vi "Handle Command.vi"(8 "error in (no error)":errorcluster, 9 "Data":variant, 10 "Command":string, 11 "Example Instrument in":refnum<class "Instrument.Element2.lvclass">) -> (0 "error out":errorcluster, 1 "Processed Data":variant, 2 "Command":string, 3 "Example Instrument out":refnum<class "Instrument.Element2.lvclass">)   [LabVIEW 2019, in "Instrument.Element2.lvclass"]
uses:
  Instrument.Element2.lvclass
  537bce52-1556-4e80-bd1c-c7a4a9f398bb.vi
  29a2691b-054e-4a4e-beb1-253e02bda3af.vi
  59852270-7c69-4675-bfeb-e3c756fddd99.vi
  537bce52-1556-4e80-bd1c-c7a4a9f398bb.vi/cb4d4a81-1a0b-4a34-ba5f-4adbbd4c364d.vi
  537bce52-1556-4e80-bd1c-c7a4a9f398bb.vi/c7ebcf92-25f2-4bb9-8687-30e4771393b5.vi
  29a2691b-054e-4a4e-beb1-253e02bda3af.vi/ce10c08f-31f2-4d71-8816-27111e331727.vi
  29a2691b-054e-4a4e-beb1-253e02bda3af.vi/b0a342ce-c0c6-4751-9e7d-832a740cbd2c.vi
  59852270-7c69-4675-bfeb-e3c756fddd99.vi/d4115e51-0f20-4ace-a191-9b88fbaefa4e.vi
  59852270-7c69-4675-bfeb-e3c756fddd99.vi/2ebf8451-a15d-4a57-978f-c6fd804eee3c.vi
  <vilib>/Utility/Data Type/Get Type Information.vi
  <vilib>/JDP Science/JSONtext/JSON text to Variant.vi
  <vilib>/JDP Science/JSONtext/LVClass Serializer/JSONtext LVClass Serializer.lvclass
  <userlib>/LevyLab/Instrument Framework/Instrument Types/VSource/Instrument.VSource.lvclass
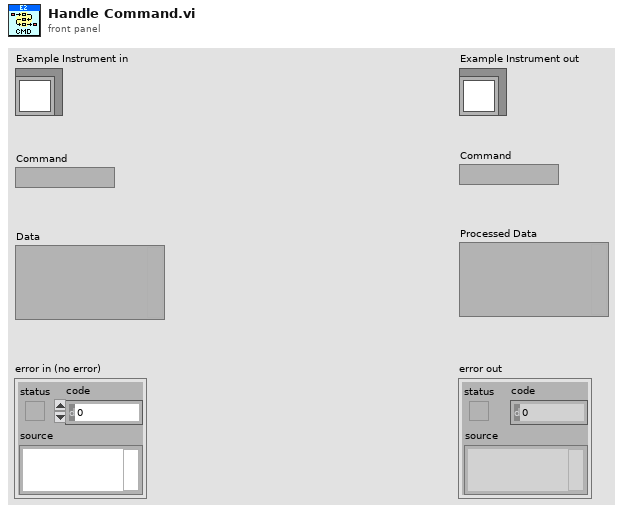
[diagram p1: front panel]
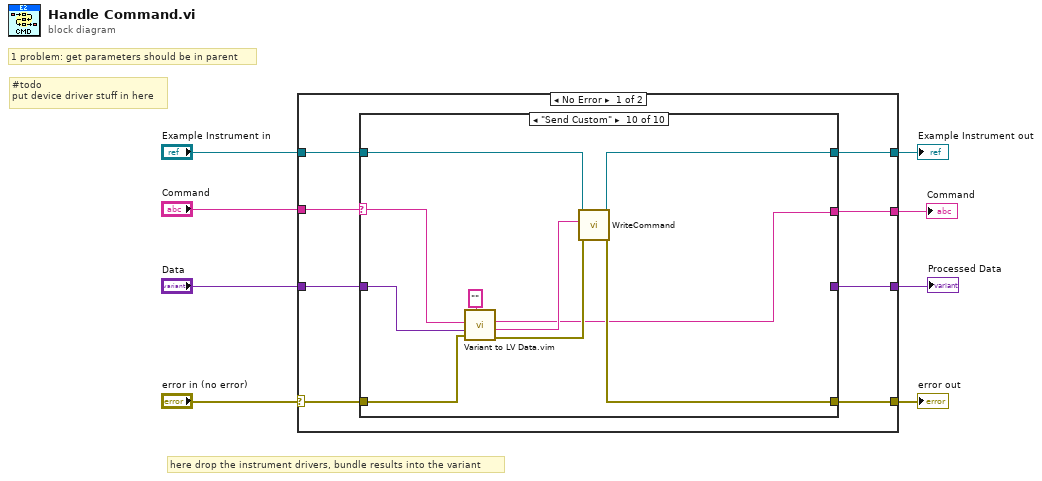
[diagram p0: block diagram]
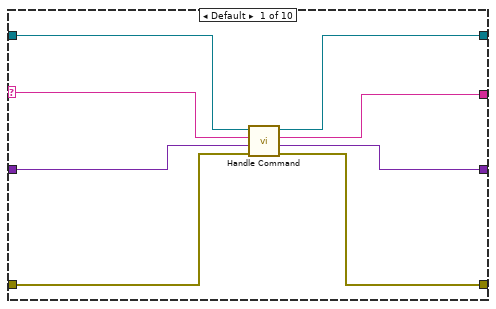
[diagram p2: hidden frame]
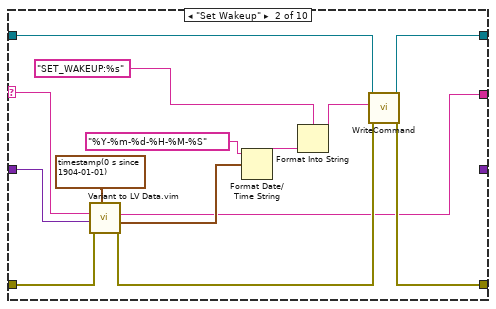
[diagram p3: hidden frame]
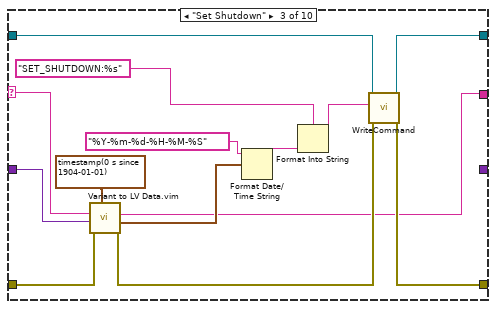
[diagram p4: hidden frame]
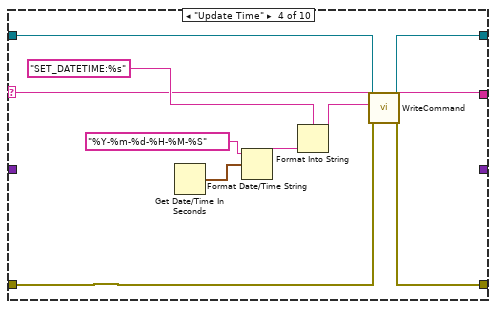
[diagram p5: hidden frame]
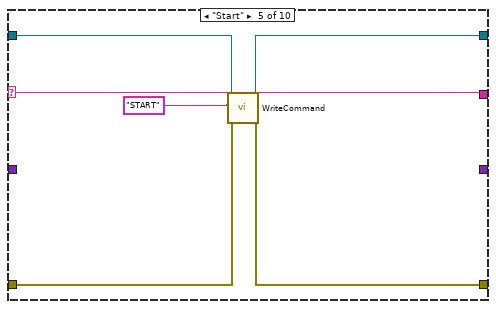
[diagram p6: hidden frame]
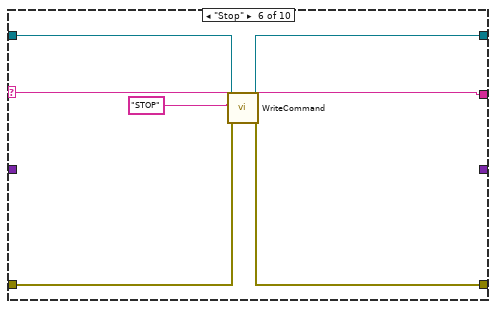
[diagram p7: hidden frame]
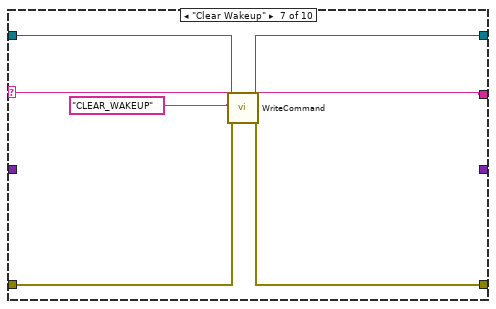
[diagram p8: hidden frame]
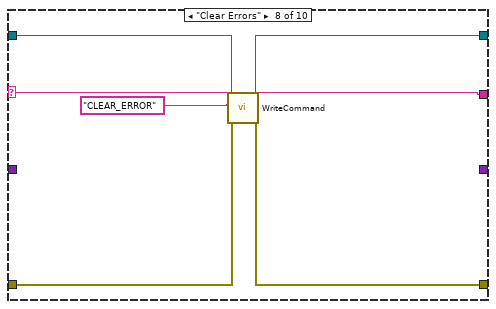
[diagram p9: hidden frame]
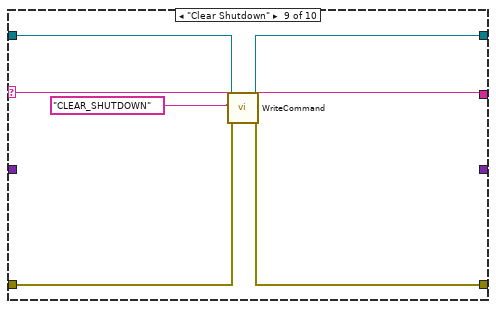
[diagram p10: hidden frame]
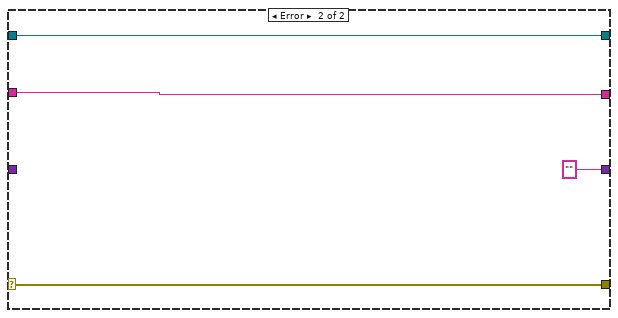
[diagram p11: hidden frame]
diagram:
  # "here drop the instrument drivers, bundle results into the variant"
  # "1 problem: get parameters should be in parent"
  # "#todo\nput device driver stuff in here"
  n1 = case shown="No Error" "error in (no error)" {
    selector: "error in (no error)" -> [w12 w106]
    tunnel: [w10 w106] -> w6
    tunnel: [w14 w105] -> w5
    tunnel: "Example Instrument in" -> [w15 w105]
    tunnel: "Command" -> [w16 w103]
    tunnel: [w13 "" ("String")] -> w3
    tunnel: "Data" -> [w11 _]
    tunnel: [w9 w103] -> w1
    frame No Error {
      n2 = case shown="\"Send Custom\"" w16 {
        selector: w16 -> [w24 w29 w43 w53 w63 w69 w75 w81 w87 w98]
        tunnel: w15 -> [w21 w38 w52 w62 w68 w74 w80 w86 w92 w102]
        tunnel: [w18 w37 w51 w61 w67 w73 w79 w85 w91 w101] -> w14
        tunnel: [w20 _ _ _ _ _ _ _ _ _] -> w13
        tunnel: w12 -> [w22 w28 w42 w55 w65 w71 w77 w83 w89 w97]
        tunnel: w11 -> [w23 w32 w46 _ _ _ _ _ _ w99]
        tunnel: [w19 w26 w40 w56 w66 w72 w78 w84 w90 w100] -> w10
        tunnel: [w17 w25 w39 w53 w63 w69 w75 w81 w87 w93] -> w9
        frame Default {
          n3 = call-parent "Handle Command.vi"("error in (no error)"=w22, "Data"=w23, "Command"=w24, "Instrument in"=w21) -> ("error out"=w19:errorcluster, "Processed Data"=w20:variant, "Command"=w17:string, "Instrument out"=w18:refnum<class "Instrument.Element2.lvclass">)  [unwired: 4 in]
        }
        frame "Set Wakeup" {
          n4 = call "Variant to LV Data.vim"("type"=timestamp(0 s since 1904-01-01) ("time stamp"), "error in (no error)"=w28, "JSON Data in"=w32, "Command"=w29) -> ("error out"=w27:errorcluster, "Data out"=w30:timestamp, "Command out"=w25:string)  [unwired: 4 in, 1 out]
          n5 = Format Date/Time String(time format string (%c)="%Y-%m-%d-%H-%M-%S", seconds (now)=w30) -> (date/time string=w35:string)  [unwired: 1 in]
          n6 = Format Into String(format string="SET_WAKEUP:%s" ("string"), w35) -> (resulting string=w33:string)  [unwired: 2 in, 1 out]
          n7 = call "WriteCommand.vi"("error in (no error)"=w27, "Command"=w33, "Instrument.Element2 in"=w38) -> ("error out"=w26:errorcluster, "Instrument.Element2 out"=w37:refnum<class "Instrument.Element2.lvclass">)  [unwired: 6 in, 1 out]
        }
        frame "Set Shutdown" {
          n8 = call "Variant to LV Data.vim"("type"=timestamp(0 s since 1904-01-01) ("time stamp"), "error in (no error)"=w42, "JSON Data in"=w46, "Command"=w43) -> ("error out"=w41:errorcluster, "Data out"=w44:timestamp, "Command out"=w39:string)  [unwired: 4 in, 1 out]
          n9 = Format Date/Time String(time format string (%c)="%Y-%m-%d-%H-%M-%S", seconds (now)=w44) -> (date/time string=w49:string)  [unwired: 1 in]
          n10 = Format Into String(format string="SET_SHUTDOWN:%s" ("string"), w49) -> (resulting string=w47:string)  [unwired: 2 in, 1 out]
          n11 = call "WriteCommand.vi"("error in (no error)"=w41, "Command"=w47, "Instrument.Element2 in"=w52) -> ("error out"=w40:errorcluster, "Instrument.Element2 out"=w51:refnum<class "Instrument.Element2.lvclass">)  [unwired: 6 in, 1 out]
        }
        frame "Update Time" {
          n12 = Get Date/Time In Seconds() -> (seconds since 1Jan1904=w54:timestamp)
          n13 = Format Date/Time String(time format string (%c)="%Y-%m-%d-%H-%M-%S", seconds (now)=w54) -> (date/time string=w59:string)  [unwired: 1 in]
          n14 = Format Into String(format string="SET_DATETIME:%s" ("string"), w59) -> (resulting string=w57:string)  [unwired: 2 in, 1 out]
          n15 = call "WriteCommand.vi"("error in (no error)"=w55, "Command"=w57, "Instrument.Element2 in"=w62) -> ("error out"=w56:errorcluster, "Instrument.Element2 out"=w61:refnum<class "Instrument.Element2.lvclass">)  [unwired: 6 in, 1 out]
        }
        frame "Start" {
          n16 = call "WriteCommand.vi"("error in (no error)"=w65, "Command"="START" ("string"), "Instrument.Element2 in"=w68) -> ("error out"=w66:errorcluster, "Instrument.Element2 out"=w67:refnum<class "Instrument.Element2.lvclass">)  [unwired: 6 in, 1 out]
        }
        frame "Stop" {
          n17 = call "WriteCommand.vi"("error in (no error)"=w71, "Command"="STOP" ("string"), "Instrument.Element2 in"=w74) -> ("error out"=w72:errorcluster, "Instrument.Element2 out"=w73:refnum<class "Instrument.Element2.lvclass">)  [unwired: 6 in, 1 out]
        }
        frame "Clear Wakeup" {
          n18 = call "WriteCommand.vi"("error in (no error)"=w77, "Command"="CLEAR_WAKEUP" ("string"), "Instrument.Element2 in"=w80) -> ("error out"=w78:errorcluster, "Instrument.Element2 out"=w79:refnum<class "Instrument.Element2.lvclass">)  [unwired: 6 in, 1 out]
        }
        frame "Clear Errors" {
          n19 = call "WriteCommand.vi"("error in (no error)"=w83, "Command"="CLEAR_ERROR" ("string"), "Instrument.Element2 in"=w86) -> ("error out"=w84:errorcluster, "Instrument.Element2 out"=w85:refnum<class "Instrument.Element2.lvclass">)  [unwired: 6 in, 1 out]
        }
        frame "Clear Shutdown" {
          n20 = call "WriteCommand.vi"("error in (no error)"=w89, "Command"="CLEAR_SHUTDOWN" ("string"), "Instrument.Element2 in"=w92) -> ("error out"=w90:errorcluster, "Instrument.Element2 out"=w91:refnum<class "Instrument.Element2.lvclass">)  [unwired: 6 in, 1 out]
        }
        frame "Send Custom" {
          n21 = call "Variant to LV Data.vim"("type"="" ("string"), "error in (no error)"=w97, "JSON Data in"=w99, "Command"=w98) -> ("error out"=w96:errorcluster, "Data out"=w94:string, "Command out"=w93:string)  [unwired: 4 in, 1 out]
          n22 = call "WriteCommand.vi"("error in (no error)"=w96, "Command"=w94, "Instrument.Element2 in"=w102) -> ("error out"=w100:errorcluster, "Instrument.Element2 out"=w101:refnum<class "Instrument.Element2.lvclass">)  [unwired: 6 in, 1 out]
        }
      }
    }
    frame Error {
    }
  }
  "error out" <- w6
  "Example Instrument out" <- w5
  "Command" <- w1
  "Processed Data" <- w3
